vi "Room Voice Switch.vi"() -> ()   [LabVIEW 2011]
uses:
  <vilib>/Analysis/NI_AALBase.lvlib
panel:
  out "Room1":bool
  out "String":string
  out "Data":dynamicdata(graph)
  out "Room2":bool
  in  "stop":bool
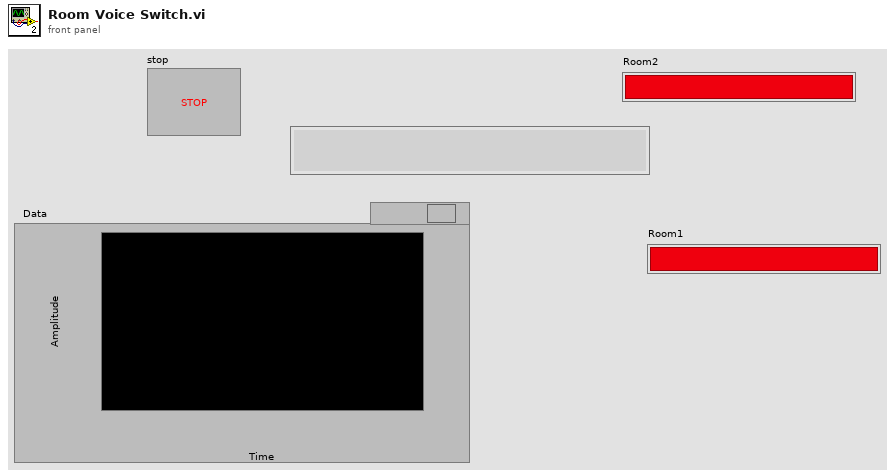
[diagram p1: front panel]
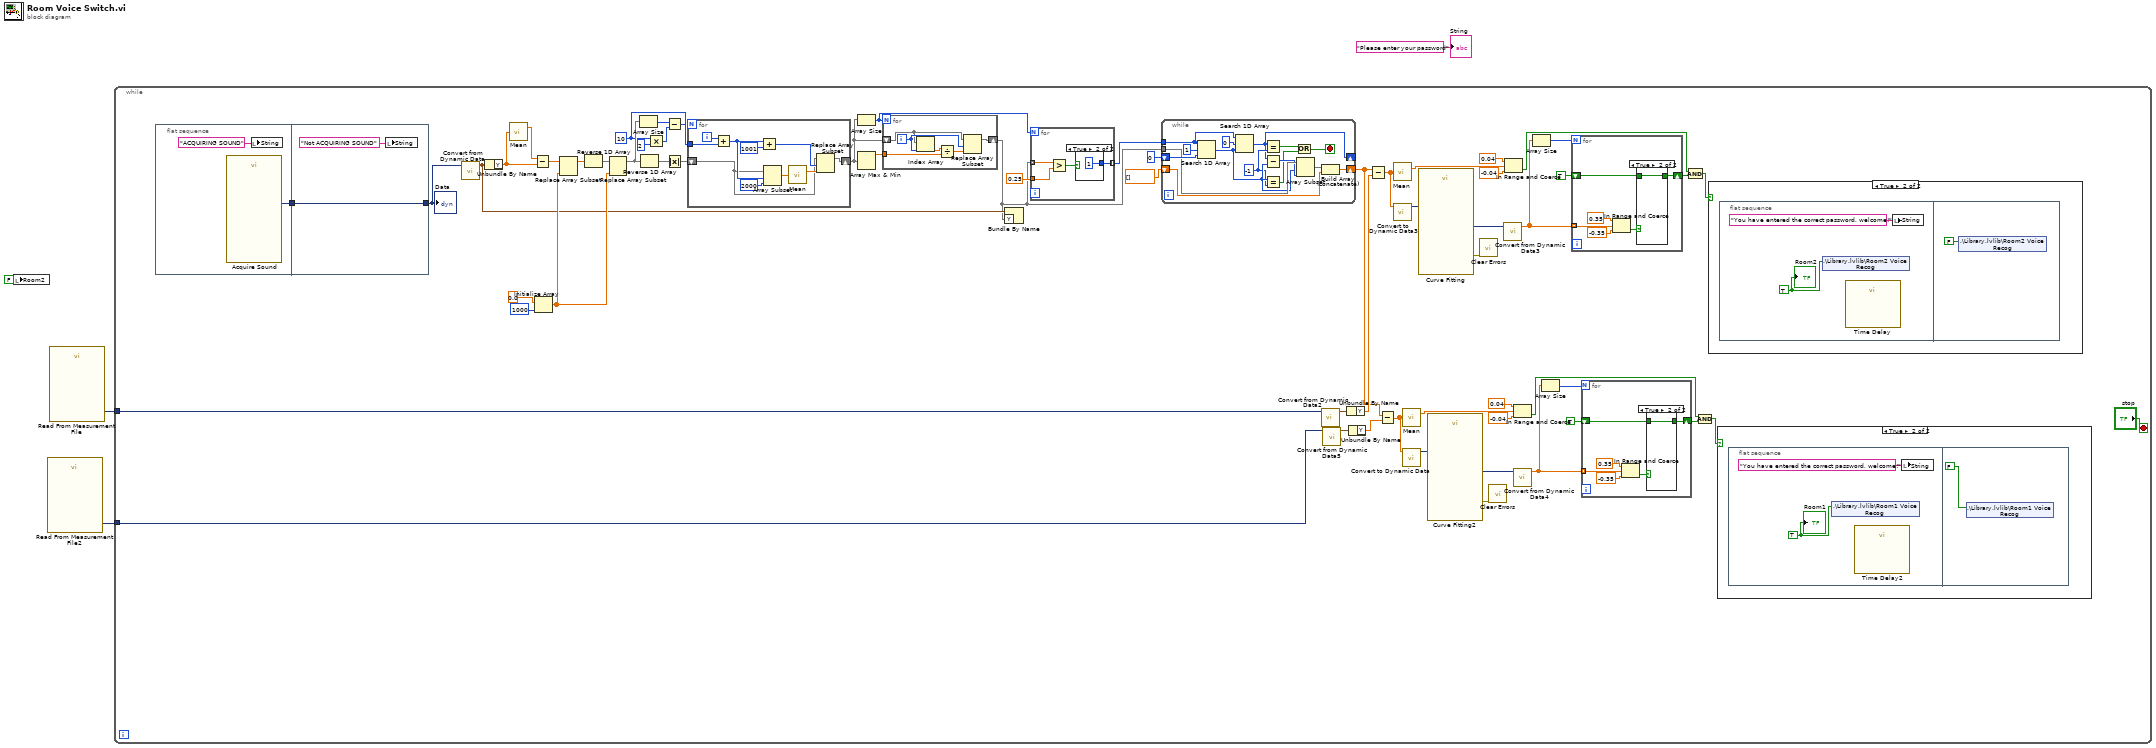
[diagram p0: block diagram]
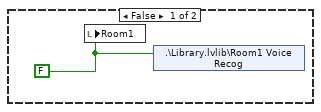
[diagram p2: hidden frame]
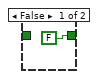
[diagram p3: hidden frame]
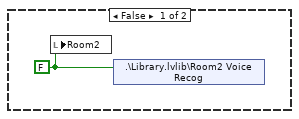
[diagram p4: hidden frame]
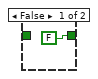
[diagram p5: hidden frame]
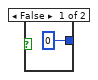
[diagram p6: hidden frame]
diagram:
  n1 = local write "Room2"(FALSE ("Led")) -> ()
  n2 = call "Read From Measurement File2"() -> ("Signals"=w1:dynamicdata)  [unwired: 6 in, 5 out]
  n3 = call "Read From Measurement File"() -> ("Signals"=w2:dynamicdata)  [unwired: 6 in, 5 out]
  n4 = while {
    tunnel: w2 -> [w65]
    tunnel: w1 -> [w6]
    stop <- "stop" stop-if-true
    w53 = 10 ("y")
    n5 = flat-sequence {
      tunnel: [w79] -> w63
      tunnel: [w81] -> w43
      tunnel: w63 -> [w81]
      frame #0 {
        n6 = call "Acquire Sound"() -> ("Data"=w79:dynamicdata)  [unwired: 18 in, 1 out]
        n7 = local write "String"("ACQUIRING SOUND" ("String")) -> ()
      }
      frame #1 {
        n8 = local write "String"("Not ACQUIRING SOUND" ("String")) -> ()
      }
    }
    n9 = call "Convert from Dynamic Data"("Dynamic Data Type"=w43) -> ("Waveform"=w39:waveform(dbl))  [unwired: 3 in]
    n10 = Unbundle By Name(w39) -> ("Y"=w41:dbl[])
    n11 = call <vilib>:"Mean.vi"("X"=w41) -> ("mean"=w42:dbl)  [unwired: 1 out]
    n12 = Subtract(x=w42, y=w41) -> (x-y=w40:dbl[])
    n13 = Initialize Array(0.0 ("element"), 1000 ("dimension size")) -> (w58:dbl[])
    n14 = Replace Array Subset(array=w40, new element=w58) -> (w60:dbl[])  [unwired: 1 in]
    n15 = Reverse 1D Array(array=w60) -> (reversed array=w59:dbl[])
    n16 = Replace Array Subset(array=w59, new element=w58) -> (w55:dbl[])  [unwired: 1 in]
    n17 = Array Size(array=w55) -> (size(s)=w54:i32)
    n18 = Reverse 1D Array(array=w55) -> (reversed array=w57:dbl[])
    n19 = Multiply(x=w53, y=2) -> (x*y=w51:i32)
    n20 = Subtract(x=w54, y=w51) -> (x-y=w50:i32)
    n21 = Absolute Value(x=w57) -> (abs(x)=w56:dbl[])
    n22 = for {
      N: w50 -> [_]
      shift-right: [w122] -> w49
      shift-left: w56 -> [w123]
      tunnel: w53 -> [w121]
      i -> [w130]
      n23 = Add(x=w130, y=w121) -> (x+y=w126:i32)
      n24 = Add(x=w126, y=1001) -> (x+y=w124:i32)
      n25 = Array Subset(array=w123, index=w126, length=2000) -> (w128:dbl[])
      n26 = call <vilib>:"Mean.vi"("X"=w128) -> ("mean"=w127:dbl)  [unwired: 1 out]
      n27 = Replace Array Subset(array=w123, new element=w127, index=w124) -> (w122:dbl[])
    }
    n28 = Array Size(array=w49) -> (size(s)=w47:i32)
    n29 = Array Max & Min(array=w49) -> (max value=w48:dbl)  [unwired: 3 out]
    n30 = for {
      N: w47 -> [_]
      tunnel: w48 -> [w117]
      shift-right: [w115] -> w38
      shift-left: w49 -> [w119]
      i -> [w120]
      n31 = Index Array(array=w119, index=w120) -> (element=w118:dbl)
      n32 = Divide(x=w118, y=w117) -> (x/y=w116:dbl)
      n33 = Replace Array Subset(array=w119, new element=w116, index=w120) -> (w115:dbl[])
    }
    n34 = Bundle By Name(cluster=w39, "Y"=w38) -> ()  [unwired: 1 out]
    n35 = for {
      N: w47 -> [_]
      tunnel: w38 -> [w112] mode=indexing
      tunnel: 0.25 -> [w111]
      tunnel: [w109] -> w37 mode=indexing
      n36 = Greater?(x=w112, y=w111) -> (0:w110:bool)
      n37 = case shown="True" w110 {
        tunnel: [0 1] -> w109
        frame False {
        }
        frame True {
        }
      }
    }
    n38 = while {
      tunnel: w37 -> [w106]
      tunnel: w38 -> [w104]
      shift-right: [w95] -> w5
      shift-left: dbl[] [] -> [w96]
      shift-right: [w94] -> _
      shift-left: 0 ("element") -> [w107]
      stop <- w98 stop-if-true
      w101 = -1 ("y")
      n39 = Search 1D Array(1D array=w106, element=1, start index (0)=w107) -> (index of element=w102:i32)
      n40 = Search 1D Array(1D array=w106, element=0, start index (0)=w102) -> (index of element=w94:i32)
      n41 = Equal?(x=w94, y=w101) -> (x = y?=w100:bool)
      n42 = Subtract(x=w94, y=w102) -> (x-y=w103:i32)
      n43 = Equal?(x=w102, y=w101) -> (x = y?=w99:bool)
      n44 = Or(x=w100, y=w99) -> (x .or. y?=w98:bool)
      n45 = Array Subset(array=w104, index=w102, length=w103) -> (w97:dbl[])
      n46 = Build Array (concatenate)(w97, w96) -> (w95:dbl[])
    }
    n47 = call "Convert from Dynamic Data2"("Dynamic Data Type"=w65) -> ("Waveform"=w36:waveform(dbl))  [unwired: 3 in]
    n48 = call "Convert from Dynamic Data5"("Dynamic Data Type"=w6) -> ("Waveform"=w8:waveform(dbl))  [unwired: 3 in]
    n49 = Unbundle By Name(w36) -> ("Y"=w35:dbl[])
    n50 = Unbundle By Name(w8) -> ("Y"=w7:dbl[])
    n51 = Subtract(x=w5, y=w35) -> (x-y=w24:dbl[])
    n52 = Subtract(x=w5, y=w7) -> (x-y=w19:dbl[])
    n53 = call <vilib>:"Mean.vi"("X"=w24) -> ("mean"=w23:dbl)  [unwired: 1 out]
    n54 = call "Convert to Dynamic Data3"("Array"=w24) -> ("Dynamic Data Type"=w28:dynamicdata)  [unwired: 3 in]
    n55 = call <vilib>:"Mean.vi"("X"=w19) -> ("mean"=w20:dbl)  [unwired: 1 out]
    n56 = call "Convert to Dynamic Data"("Array"=w19) -> ("Dynamic Data Type"=w15:dynamicdata)  [unwired: 3 in]
    n57 = call "Curve Fitting"("Signals"=w28) -> ("error out"=w22:errorcluster, "best fit"=w27:dynamicdata)  [unwired: 7 in, 2 out]
    n58 = call "Curve Fitting2"("Signals"=w15) -> ("error out"=w21:errorcluster, "best fit"=w16:dynamicdata)  [unwired: 7 in, 2 out]
    n59 = call <vilib>:"Clear Errors.vi"("error in (no error)"=w22) -> ()  [unwired: 6 in, 1 out]
    n60 = call <vilib>:"Clear Errors.vi"("error in (no error)"=w21) -> ()  [unwired: 6 in, 1 out]
    n61 = call "Convert from Dynamic Data3"("Dynamic Data Type"=w27) -> ("Array"=w26:dbl[])  [unwired: 3 in]
    n62 = In Range and Coerce(upper limit=0.04, x=w23, lower limit=-0.04) -> (In Range?=w31:bool)  [unwired: 1 out]
    n63 = call "Convert from Dynamic Data4"("Dynamic Data Type"=w16) -> ("Array"=w17:dbl[])  [unwired: 3 in]
    n64 = In Range and Coerce(upper limit=0.04, x=w20, lower limit=-0.04) -> (In Range?=w12:bool)  [unwired: 1 out]
    n65 = Array Size(array=w26) -> (size(s)=w29:i32)
    n66 = Array Size(array=w17) -> (size(s)=w14:i32)
    n67 = for {
      N: w29 -> [_]
      tunnel: w26 -> [w91] mode=indexing
      shift-right: [w86] -> w30
      shift-left: TRUE -> [w87]
      n68 = In Range and Coerce(upper limit=0.35, x=w91, lower limit=-0.35) -> (In Range?=w88:bool)  [unwired: 1 out]
      n69 = case shown="True" w88 {
        tunnel: [FALSE w93] -> w86
        tunnel: w87 -> [_ w93]
        frame False {
        }
        frame True {
        }
      }
    }
    n70 = for {
      N: w14 -> [_]
      tunnel: w17 -> [w75] mode=indexing
      shift-right: [w70] -> w13
      shift-left: TRUE -> [w71]
      n71 = In Range and Coerce(upper limit=0.35, x=w75, lower limit=-0.35) -> (In Range?=w72:bool)  [unwired: 1 out]
      n72 = case shown="True" w72 {
        tunnel: [FALSE w77] -> w70
        tunnel: w71 -> [_ w77]
        frame False {
        }
        frame True {
        }
      }
    }
    n73 = Compound Arithmetic op=AND(w31, w30) -> (w25:bool)
    n74 = Compound Arithmetic op=AND(w12, w13) -> (w18:bool)
    n75 = case shown="True" w25 {
      frame False {
        w82 = FALSE ("Led")
        n76 = local write "Room2"(w82) -> ()
        n77 = shared-variable ".\\Library.lvlib\\Room2 Voice Recog"(w82) -> ()  [unwired: 1 in, 1 out]
      }
      frame True {
        n78 = flat-sequence {
          frame #0 {
            w83 = TRUE ("Led")
            n79 = shared-variable ".\\Library.lvlib\\Room2 Voice Recog"(w83) -> ()  [unwired: 1 in, 1 out]
            n80 = call "Time Delay"() -> ()  [unwired: 11 in, 1 out]
            n81 = local write "String"("You have entered the correct password, welcome!") -> ()
            "Room2" <- w83
          }
          frame #1 {
            n82 = shared-variable ".\\Library.lvlib\\Room2 Voice Recog"(FALSE ("Room2 Voice Recog")) -> ()  [unwired: 1 in, 1 out]
          }
        }
      }
    }
    n83 = case shown="True" w18 {
      frame False {
        w66 = FALSE ("Led")
        n84 = local write "Room1"(w66) -> ()
        n85 = shared-variable ".\\Library.lvlib\\Room1 Voice Recog"(w66) -> ()  [unwired: 1 in, 1 out]
      }
      frame True {
        n86 = flat-sequence {
          frame #0 {
            w67 = TRUE ("Led")
            n87 = shared-variable ".\\Library.lvlib\\Room1 Voice Recog"(w67) -> ()  [unwired: 1 in, 1 out]
            n88 = call "Time Delay2"() -> ()  [unwired: 11 in, 1 out]
            n89 = local write "String"("You have entered the correct password, welcome!") -> ()
            "Room1" <- w67
          }
          frame #1 {
            n90 = shared-variable ".\\Library.lvlib\\Room1 Voice Recog"(FALSE ("stop")) -> ()  [unwired: 1 in, 1 out]
          }
        }
      }
    }
    "Data" <- w43
  }
  "String" <- "Please enter your password"
